vi "Position Right Pane Tab.vi"(8 "Error In":errorcluster, 11 "TabCtl Refnum":refnum<vi>) -> (0 "Error Out":errorcluster)   [LabVIEW 2014]
uses:
  <vilib>/Utility/miscctls.llb/LVPositionTypeDef.ctl
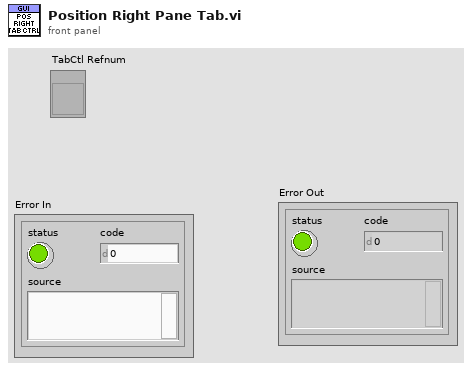
[diagram p1: front panel]
types:
  T1 = typedef "LVPositionTypeDef.ctl" = cluster{"Left":i32, "Top":i32}
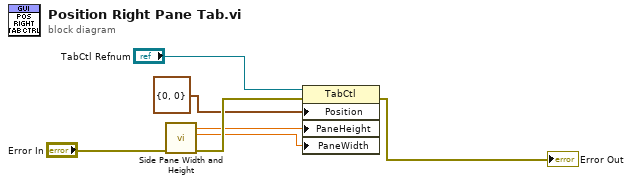
[diagram p0: block diagram]
diagram:
  n1 = call "Side Pane Width and Height.vi"("error in (no error)"="Error In") -> ("error out"=w5:errorcluster, "Width"=w2:dbl, "Height"=w3:dbl)  [unwired: 8 in]
  n2 = property class="TabCtl"(reference="TabCtl Refnum", error in=w5, "Position"=T1 {"Left"=0, "Top"=0}, "PaneHeight"=w3, "PaneWidth"=w2) -> (error out=→"Error Out":errorcluster)  [unwired: 1 out]
